vi "LAChatByText.vi"(8 "Error In":errorcluster, 9 "isChunk(T)":bool=TRUE, 10 "Message":string, 11 "LiteAgent In":T1) -> (0 "Error Out":errorcluster, 3 "LiteAgent Out":T1)   [LabVIEW 2017, in "LiteAgentSDK.lvlib"]
uses:
  LiteAgentSDK.lvlib
  C:/Users/Jan/Projects/LiteAgentSDK-LabVIEW/Source/Bin/LiteAgentSDK.LabVIEW.dll
  Bin/LiteAgentSDK.LabVIEW.dll
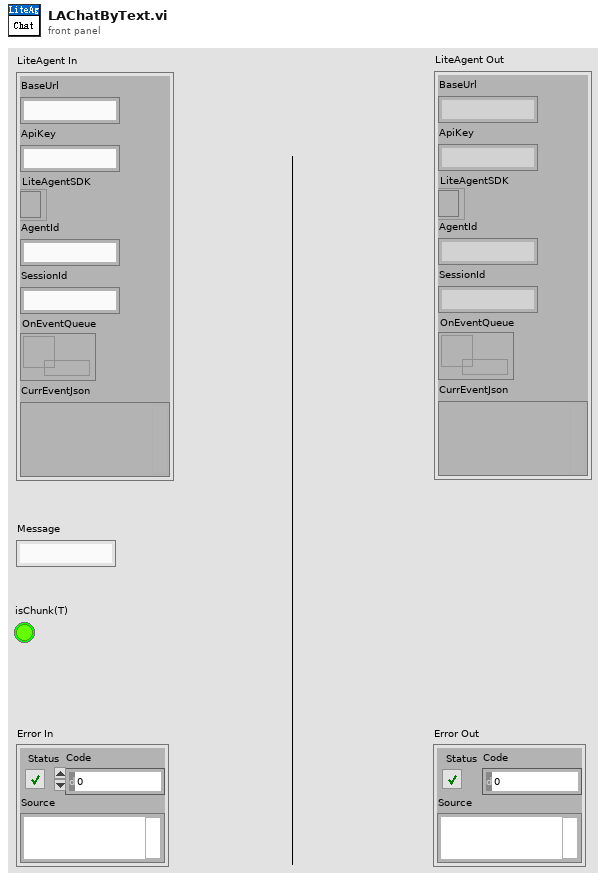
[diagram p1: front panel]
types:
  T1 = cluster{"BaseUrl":string, "ApiKey":string, "LiteAgentSDK":refnum<k24>, "AgentId":string, "SessionId":string, "OnEventQueue":refnum<queue>, "CurrEventJson":variant}
  T2 = cluster{"content":cluster{"type":string, "message":string}[], "isChunk":bool}
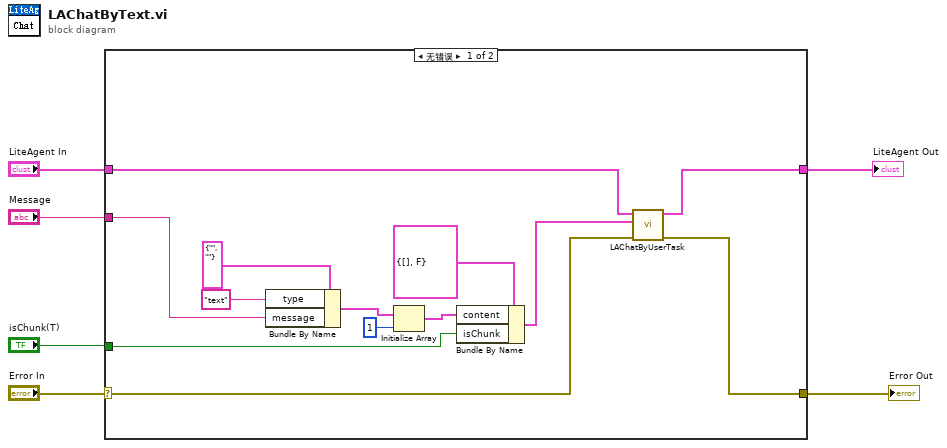
[diagram p0: block diagram]
diagram:
  n1 = case shown="无错误" "Error In" {
    selector: "Error In" -> [w11 w21]
    tunnel: [w10 w21] -> w5
    tunnel: "LiteAgent In" -> [w8 w20]
    tunnel: [w7 w20] -> w3
    tunnel: "isChunk(T)" -> [w13 _]
    tunnel: "Message" -> [w12 _]
    frame No Error {
      n2 = Bundle By Name(cluster=cluster{"type":string, "message":string} {"type"="", "message"=""} ("content"), "type"="text", "message"=w12) -> (w18:cluster{"type":string, "message":string})
      n3 = Initialize Array(w18, 1 ("维数大小")) -> (w19:cluster{"type":string, "message":string}[])
      n4 = Bundle By Name(cluster=T2 {"content"=[], "isChunk"=FALSE} ("UserTask"), "content"=w19, "isChunk"=w13) -> (w9:T2)
      n5 = call "LAChatByUserTask.vi"("Error In"=w11, "UserTask"=w9, "LiteAgent In"=w8) -> ("Error Out"=w10:errorcluster, "LiteAgent Out"=w7:T1)  [unwired: 7 in]
    }
    frame Error {
    }
  }
  "Error Out" <- w5
  "LiteAgent Out" <- w3
